vi "Test Port Reading.vi"(8 "error in (no error)":errorcluster, 11 "TestCase in":refnum<class "LecturaADC.lvclass">) -> (0 "error out":errorcluster, 3 "TestCase out":refnum<class "LecturaADC.lvclass">)   [LabVIEW 2020, in "LecturaADC.lvclass"]
uses:
  LecturaADC.lvclass
  Simulated Device/Simulated Device.lvclass
  <vilib>/addons/_JKI Toolkits/VI Tester/TestCase.llb/TestCase.lvclass
  C:/Program Files (x86)/National Instruments/LabVIEW 2020/vi.lib/addons/_JKI Toolkits/VI Tester/TestCase.llb/TestCase.lvclass
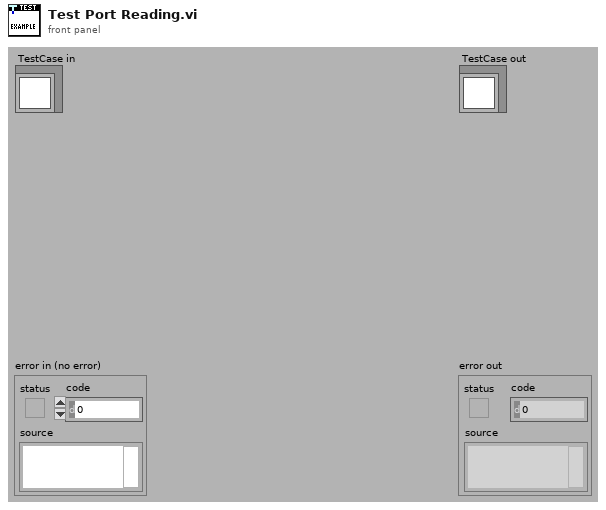
[diagram p1: front panel]
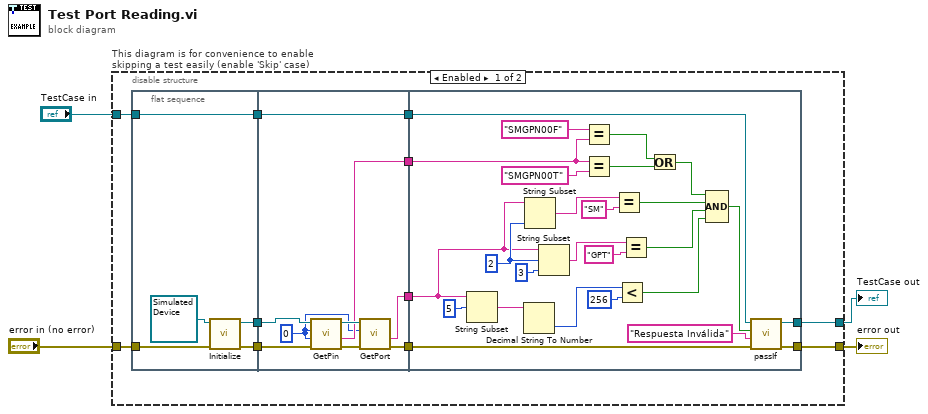
[diagram p0: block diagram]
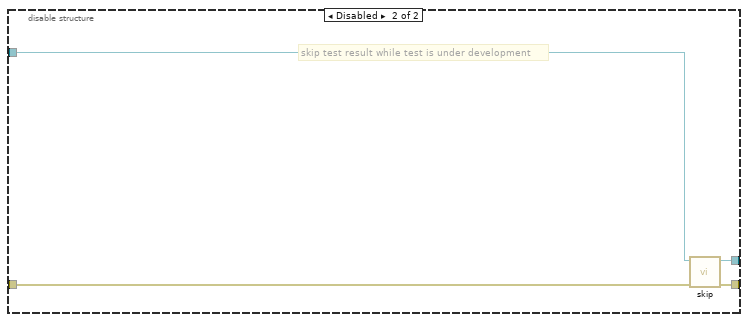
[diagram p2: hidden frame]
diagram:
  n1 = disable-structure "This diagram is for convenience to enable skipping a test easily (enable 'Skip' case)" shown="Enabled" {
    disable-tunnel: "TestCase in" -> [w15 w59]
    disable-tunnel: [w12 w57] -> w1
    disable-tunnel: [w13 w58] -> w3
    disable-tunnel: "error in (no error)" -> [w14 w56]
    frame Enabled {
      n2 = flat-sequence {
        tunnel: w15 -> [w20]
        tunnel: w14 -> [w18]
        tunnel: [w20] -> w11
        tunnel: [w17] -> w9
        tunnel: [w16] -> w8
        tunnel: w11 -> [w29]
        tunnel: [w29] -> w10
        tunnel: w9 -> [w27]
        tunnel: w8 -> [w28]
        tunnel: [w24] -> w7
        tunnel: [w23] -> w6
        tunnel: [w21] -> w5
        tunnel: [w55] -> w13
        tunnel: [w54] -> w12
        tunnel: w10 -> [w53]
        tunnel: w7 -> [w52]
        tunnel: w6 -> [w36]
        tunnel: w5 -> [w38]
        frame #0 {
          n3 = call-dynamic "Initialize.vi"("error in (no error)"=w18, "Simulated Device in"=refnum<class "Simulated Device.lvclass"> refnum ("Simulated Device.lvclass")) -> ("error out"=w17:errorcluster, "Simulated Device out"=w16:refnum<class "Simulated Device.lvclass">)  [unwired: 7 in, 1 out]
        }
        frame #1 {
          w22 = u8 0 ("Port")
          n4 = call-dynamic "GetPin.vi"("error in (no error)"=w27, "Pin"=w22, "Port"=w22, "Simulated Device in"=w28) -> ("error out"=w26:errorcluster, "Response"=w23:string, "Simulated Device out"=w25:refnum<class "Simulated Device.lvclass">)  [unwired: 4 in, 1 out]
          n5 = call-dynamic "GetPort.vi"("error in (no error)"=w26, "Port"=w22, "Simulated Device in"=w25) -> ("error out"=w24:errorcluster, "Response"=w21:string)  [unwired: 5 in, 2 out]
        }
        frame #2 {
          w51 = 2 ("length (rest)")
          n6 = String Subset(string=w38, offset (0)=5) -> (substring=w44:string)  [unwired: 1 in]
          n7 = Decimal String To Number(string=w44) -> (number=w43:i32)  [unwired: 2 in, 1 out]
          n8 = String Subset(string=w38, length (rest)=w51) -> (substring=w48:string)  [unwired: 1 in]
          n9 = String Subset(string=w38, offset (0)=w51, length (rest)=3 ("length (rest)")) -> (substring=w46:string)
          n10 = Equal?(x="SMGPN00F" ("y"), y=w36) -> (x = y?=w34:bool)
          n11 = Equal?(x=w36, y="SMGPN00T") -> (x = y?=w33:bool)
          n12 = Equal?(x=w48, y="SM") -> (x = y?=w41:bool)
          n13 = Less?(x=w43, y=256) -> (x < y?=w39:bool)
          n14 = Equal?(x=w46, y="GPT") -> (x = y?=w40:bool)
          n15 = Or(x=w34, y=w33) -> (x .or. y?=w32:bool)
          n16 = Compound Arithmetic op=AND(w32, w41, w40, w39) -> (w31:bool)
          n17 = call-dynamic "passIf.vi"("error in (no error)"=w52, "message (\"\")"="Respuesta Inválida" ("message (\"\")"), "pass"=w31, "TestCase in"=w53) -> ("error out"=w55:errorcluster, "TestCase out"=w54:refnum<class "LecturaADC.lvclass">)  [unwired: 6 in]
        }
      }
    }
    frame Disabled {
      # "skip test result while test is under development"
      n18 = call <vilib>:"skip.vi"("error in (no error)"=w56, "TestCase in"=w59) -> ("error out"=w58:errorcluster, "TestCase out"=w57:refnum<class "LecturaADC.lvclass">)  [unwired: 8 in]
    }
  }
  "error out" <- w3
  "TestCase out" <- w1
